vi "IsColliding.vi"(1 "RobotRef":refnum<class "Robot.lvclass">[](array[class]), 4 "RobotRadius":dbl, 5 "error in (no error)":errorcluster) -> (15 "IsCollinding":bool, 19 "error out":errorcluster)   [LabVIEW 2024, in "DefendAreaTactic.lvclass"]
uses:
  DefendAreaTactic.lvclass
  Robot_class/Robot.lvclass
  Robot_class/Robot.lvclass/Robot.ctl
  Robot_class/Read dest_x.vi
  Robot_class/Read dest_y.vi
  Utilities_class/Utilities.lvclass
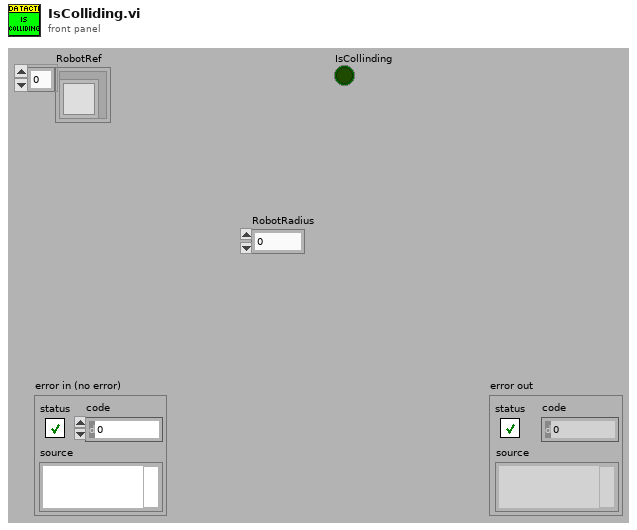
[diagram p1: front panel]
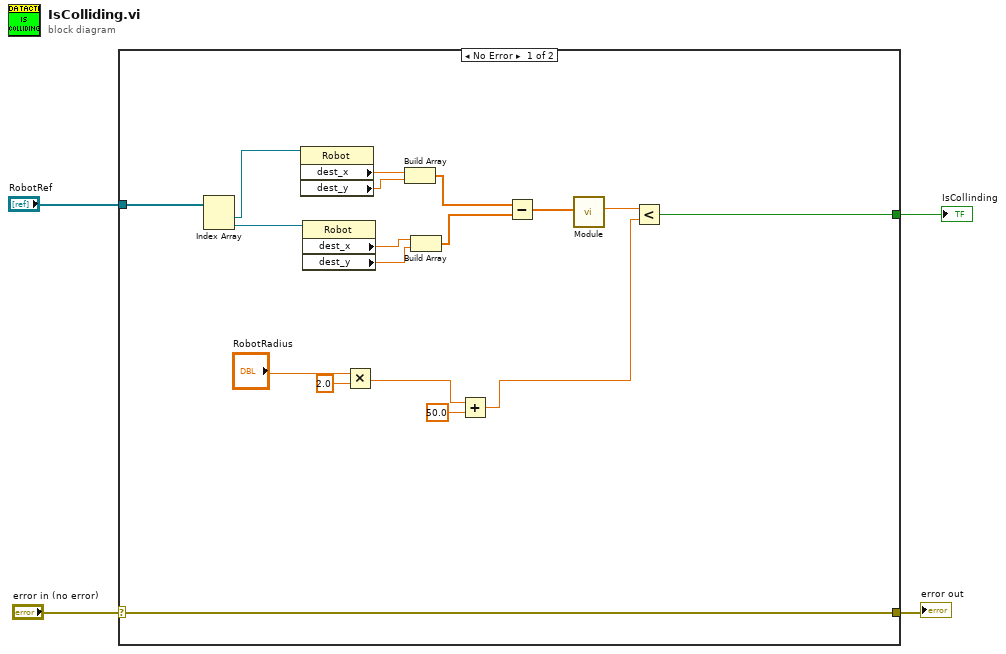
[diagram p0: block diagram]
diagram:
  n1 = case shown="No Error" "error in (no error)" {
    selector: "error in (no error)" -> [w22 w23]
    tunnel: [w22 w23] -> w3
    tunnel: "RobotRef" -> [w21 _]
    tunnel: [w10 _] -> w1
    frame No Error {
      n2 = Index Array(array=w21) -> (element #1=w20:refnum<class "Robot.lvclass">, element #2=w19:refnum<class "Robot.lvclass">)  [unwired: 2 in]
      n3 = property class="Robot"(reference=w20) -> ("dest_x"=w18:dbl, "dest_y"=w17:dbl)  [unwired: 1 in, 2 out]
      n4 = property class="Robot"(reference=w19) -> ("dest_x"=w16:dbl, "dest_y"=w15:dbl)  [unwired: 1 in, 2 out]
      n5 = Multiply(x="RobotRadius", y=2.0) -> (x*y=w6:dbl)
      n6 = Build Array(w18, w17) -> (w14:dbl[])
      n7 = Build Array(w16, w15) -> (w13:dbl[])
      n8 = Add(x=w6, y=50.0) -> (x+y=w5:dbl)
      n9 = Subtract(x=w14, y=w13) -> (x-y=w12:dbl[])
      n10 = call "Module.vi"("2D vector"=w12) -> ("Modulo"=w11:dbl)  [unwired: 8 in, 2 out]
      n11 = Less?(x=w11, y=w5) -> (x < y?=w10:bool)
    }
    frame Error {
    }
  }
  "error out" <- w3
  "IsCollinding" <- w1
